vi "Do This.vi"(8 "error in (no error)":errorcluster, 10 "Status Events":refnum<class "Status Events.lvclass">, 11 "Run VI Tester in":refnum<class "Run VI Tester.lvclass">) -> (0 "error out":errorcluster, 3 "Run VI Tester out":refnum<class "Run VI Tester.lvclass">)   [LabVIEW 2014, in "Run VI Tester.lvclass"]
uses:
  Run VI Tester.lvclass
  Shared/Classes/Status Events/Status Events.lvclass
  Classes/Job/Job.lvclass/Job.ctl
  Run VI Tester.lvclass/Run VI Tester.ctl
  <vilib>/Utility/error.llb/DialogType.ctl
  Classes/Job/Job.lvclass
  JUnit/VI Tester Parsing.lvlib
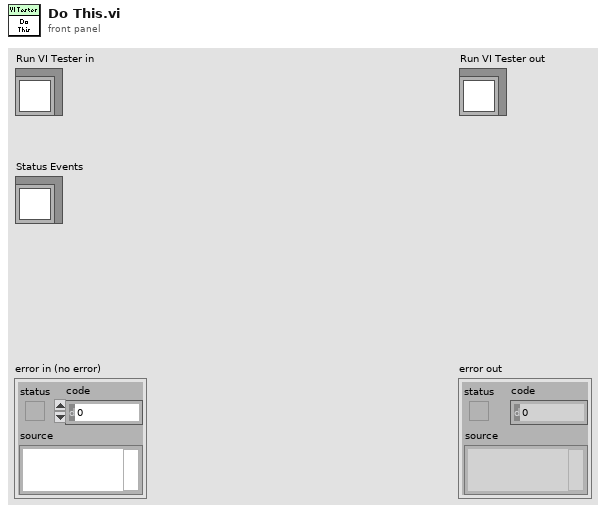
[diagram p1: front panel]
types:
  T1 = typedef "JUnit API.lvlib/Test Suite Attribute Values.ctl" = cluster{"name":string, "tests":i32, "failures":i32, "errors":i32, "time":dbl, "disabled":i32, "skipped":i32, "skips":i32, "timestamp":dbl, "hostname":string, "id":string, "package":string, "assertions":i32, "file":string, "skip":string, "log":string, "url":string}
  T2 = typedef "DialogType.ctl" = u16
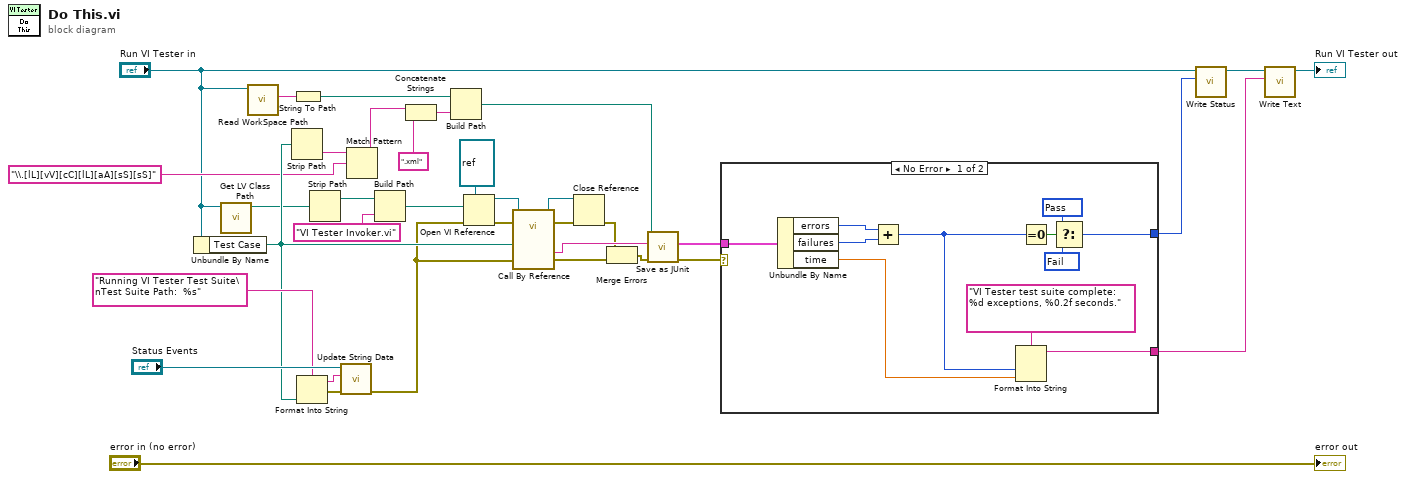
[diagram p0: block diagram]
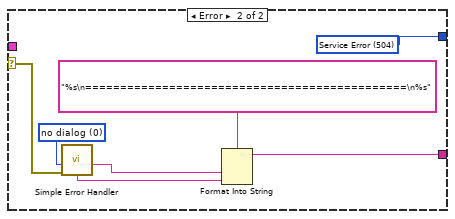
[diagram p2: hidden frame]
diagram:
  n1 = Unbundle By Name("Run VI Tester in") -> ("Test Case"=w18:path)
  n2 = call <vilib>:"Get LV Class Path.vi"("object"="Run VI Tester in") -> ("class path"=w3:path)  [unwired: 9 in, 1 out]
  n3 = call "Read WorkSpace Path.vi"("Job in"="Run VI Tester in") -> ("WorkSpace Path"=w26:string)  [unwired: 8 in, 2 out]
  n4 = Strip Path(path=w18) -> (name=w28:string)  [unwired: 1 out]
  n5 = String To Path(string=w26) -> (path=w27:path)
  n6 = Format Into String(format string="Running VI Tester Test Suite\nTest Suite Path:  %s", w18) -> (resulting string=w23:string, error out=w22:errorcluster)  [unwired: 2 in]
  n7 = Strip Path(path=w3) -> (stripped path=w2:path)  [unwired: 1 out]
  n8 = call "Update String Data.vi"("error in (no error)"=w22, "String Data"=w23, "Status Updater in"="Status Events") -> ("error out"=w17:errorcluster)  [unwired: 7 in, 1 out]
  n9 = Match Pattern(string=w28, regular expression="\\.[lL][vV][cC][lL][aA][sS][sS]") -> (before substring=w21:string)  [unwired: 1 in, 3 out]
  n10 = Build Path(base path=w2, name or relative path="VI Tester Invoker.vi") -> (appended path=w14:path)
  n11 = Concatenate Strings(w21, ".xml" ("string")) -> (w20:string)
  n12 = Build Path(base path=w27, name or relative path=w20) -> (appended path=w15:path)
  n13 = Open VI Reference(type specifier VI Refnum (for type only)=refnum<vi> refnum, vi path=w14, error in (no error)=w17) -> (vi reference=w11:refnum<vi>, error out=w13:errorcluster)  [unwired: 3 in]
  n14 = call-by-ref "?"(reference=w11, error in=w13, 8:"error in (no error)"=w17, "Test Path"=w18) -> (reference out=w10:refnum<vi>, error out=w12:errorcluster, 0:"error out"=w7:errorcluster, "test details"=w8:string)  [unwired: 7 in, 1 out]
  n15 = Close Reference(reference=w10, error in (no error)=w12) -> (error out=w5:errorcluster)
  n16 = Merge Errors(w5, w7) -> (w6:errorcluster)
  n17 = call "Save as JUnit.vi"("error in (no error)"=w6, "Raw Results String"=w8, "XML file path"=w15) -> ("error out"=w25:errorcluster, "Test Header"=w24:T1)  [unwired: 7 in]
  n18 = case shown="No Error" w25 {
    selector: w25 -> [_ w48]
    tunnel: [w40 w53] -> w30
    tunnel: [w44 w47] -> w29
    tunnel: w24 -> [w39 _]
    frame No Error {
      w42 = u16 200 items=["Service Error"=504, "Abort"=503, "Fail"=500, "Pass"=200] ("Status")
      w43 = u16 500 items=["Service Error"=504, "Abort"=503, "Fail"=500, "Pass"=200] ("Status")
      n19 = Unbundle By Name(w39) -> ("errors"=w36:i32, "failures"=w38:i32, "time"=w45:dbl)
      n20 = Add(x=w36, y=w38) -> (x+y=w37:i32)
      n21 = Format Into String(format string="VI Tester test suite complete:  %d exceptions, %0.2f seconds.", w37, w45) -> (resulting string=w44:string)  [unwired: 2 in, 1 out]
      n22 = Equal To 0?(x=w37) -> (x = 0?=w41:bool)
      n23 = Select(t=w42, s=w41, f=w43) -> (s? t:f=w40:u16)
    }
    frame Error {
      w52 = T2 0 items=["no dialog", "OK message", "continue or stop message", "OK message + warnings", "continue/stop + warnings"] ("type of dialog (OK msg:1)")
      w53 = u16 504 items=["Service Error"=504, "Abort"=503, "Fail"=500, "Pass"=200] ("Status")
      n24 = call <vilib>:"Simple Error Handler.vi"("type of dialog (OK msg:1)"=w52, "error in (no error)"=w48) -> ("source out"=w50:string, "message"=w49:string)  [unwired: 3 in, 3 out]
      n25 = Format Into String(format string="%s\n==============================================\n%s", w50, w49) -> (resulting string=w47:string)  [unwired: 2 in, 1 out]
    }
  }
  n26 = call "Write Status.vi"("Status"=w30, "Job in"="Run VI Tester in") -> ("Job out"=w35:refnum<class "Run VI Tester.lvclass">)  [unwired: 8 in, 1 out]
  n27 = call "Write Text.vi"("Text"=w29, "Job in"=w35) -> ("Job out"=→"Run VI Tester out":refnum<class "Run VI Tester.lvclass">)  [unwired: 8 in, 1 out]
  "error out" <- "error in (no error)"
